vi "SVX Buffer Waterfall Graph (Plot Array).vi"(5 "reset on change to dx (F)":bool, 6 "number of spectra (40)":i32=40, 7 "reset? (F)":bool, 8 "error in (no error)":errorcluster, 9 "dz":dbl=1.0, 10 "initial z0":dbl, 11 "plots":cluster{"x0":dbl, "dx":dbl, "Y":dbl[]}[](array[cluster])) -> (0 "error out":errorcluster, 3 "waterfall graph data out":T2={"z0"=0.0, "dz"=1.0, "plots"=[]})   [LabVIEW 2017, in "SoundVib_SpectralDisplay.lvlib"]
doc: "Buffers signals and returns the buffered signals up to a maximum count. If you use this VI with the Waterfall Graph, the display mimics the behavior of a chart. Wire data to the <B>waterfall graph data</B> input to determine the polymorphic instance to use or manually select the instance."
uses:
  <vilib>/addons/Sound and Vibration/Order Analysis/Data Presentation/SoundVib_SpectralDisplay.lvlib
panel:
  in  "waterfall graph data":T1={"z0"=0.0, "dz"=1.0, "Plots"=[]}
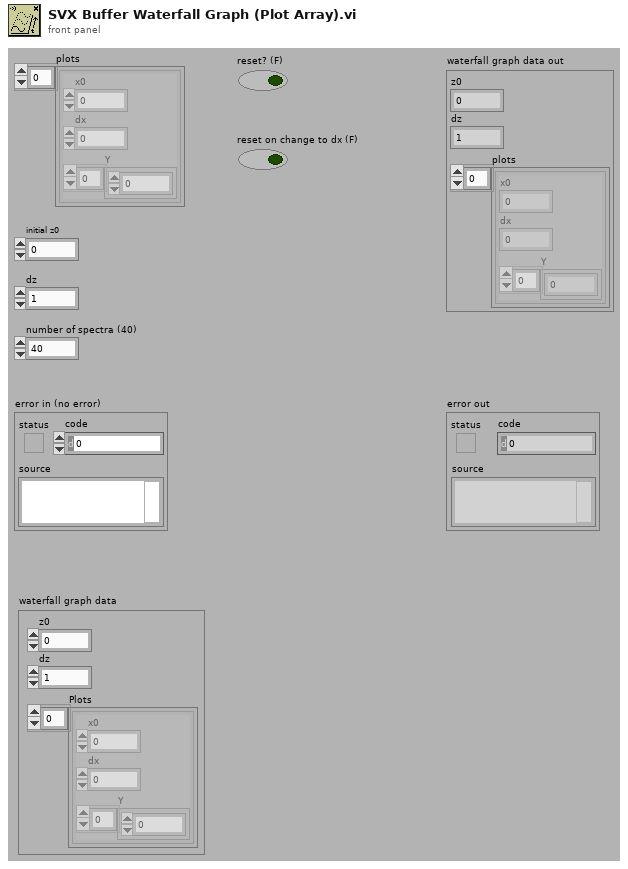
[diagram p1: front panel]
types:
  T1 = cluster{"z0":dbl, "dz":dbl, "Plots":cluster{"x0":dbl, "dx":dbl, "Y":dbl[]}[]}
  T2 = cluster{"z0":dbl, "dz":dbl, "plots":cluster{"x0":dbl, "dx":dbl, "Y":dbl[]}[]}
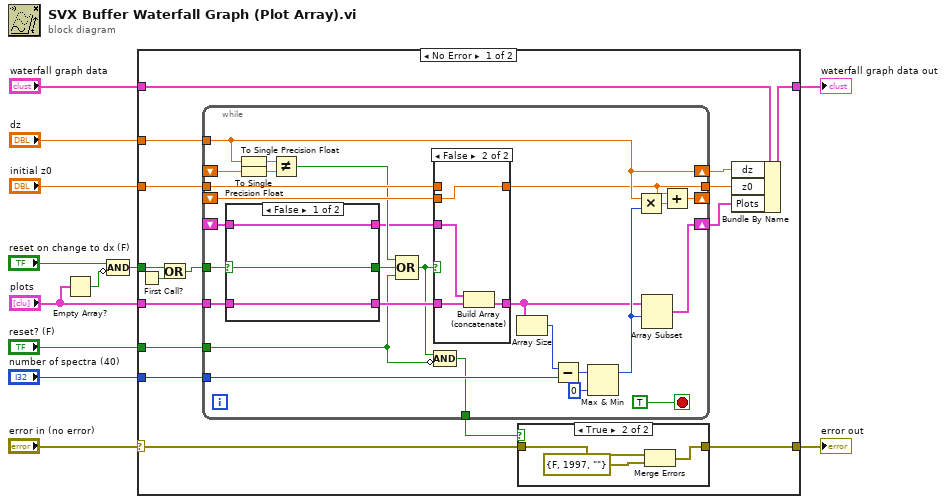
[diagram p0: block diagram]
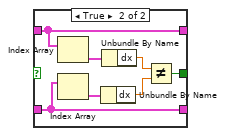
[diagram p4: hidden frame]
diagram:
  n1 = Empty Array?(array="plots") -> (empty?=w3:bool)
  n2 = Compound Arithmetic op=AND("reset on change to dx (F)", invert w3) -> (w1:bool)
  n3 = case shown="No Error" "error in (no error)" {
    selector: "error in (no error)" -> [w17 w77]
    tunnel: [w16 w77] -> w11
    tunnel: "reset? (F)" -> [w22 _]
    tunnel: "number of spectra (40)" -> [w28 _]
    tunnel: "plots" -> [w21 _]
    tunnel: [w27 w76] -> w8
    tunnel: "dz" -> [w25 _]
    tunnel: "initial z0" -> [w24 _]
    tunnel: "waterfall graph data" -> [w23 w76]
    tunnel: w1 -> [w20 _]
    frame No Error {
      n4 = First Call?() -> (First Call?: T/F=w13:bool)
      n5 = Or(x=w20, y=w13) -> (x .or. y?=w14:bool)
      n6 = while {
        tunnel: w28 -> [w41]
        shift-right: [w58] -> w26
        shift-left: _ -> [w44]
        tunnel: w22 -> [w36]
        shift-right: [w54] -> _
        shift-left: _ -> [w56]
        tunnel: w21 -> [w43]
        tunnel: w25 -> [w50]
        tunnel: w24 -> [w51]
        shift-right: [w50] -> w19
        shift-left: _ -> [w52]
        tunnel: w14 -> [w47]
        tunnel: [w35] -> w18
        tunnel: [w34] -> w15
        stop <- TRUE stop-if-true
        n7 = case shown="False" w47 {
          selector: w47 -> [w68 _]
          tunnel: w44 -> [w67 w70]
          tunnel: [w68 w73] -> w48
          tunnel: w43 -> [w66 w69]
          tunnel: [w67 w70] -> w39
          tunnel: [w66 w69] -> w40
          frame False {
          }
          frame True {
            n8 = Index Array(array=w70) -> (element=w75:cluster{"x0":dbl, "dx":dbl, "Y":dbl[]})  [unwired: 1 in]
            n9 = Index Array(array=w69) -> (element=w72:cluster{"x0":dbl, "dx":dbl, "Y":dbl[]})  [unwired: 1 in]
            n10 = Unbundle By Name(w72) -> ("dx"=w71:dbl)
            n11 = Unbundle By Name(w75) -> ("dx"=w74:dbl)
            n12 = Not Equal?(x=w74, y=w71) -> (x != y?=w73:bool)
          }
        }
        n13 = To Single Precision Float(number=w50) -> (single precision float=w45:sgl)
        n14 = To Single Precision Float(number=w52) -> (single precision float=w46:sgl)
        n15 = Not Equal?(x=w45, y=w46) -> (x != y?=w49:bool)
        n16 = Compound Arithmetic op=OR(w49, w48, w36) -> (w37:bool)
        n17 = case shown="False" w37 {
          tunnel: [w60 w62] -> w33
          tunnel: w56 -> [_ w65]
          tunnel: [w61 w65] -> w34
          tunnel: w51 -> [w61 _]
          tunnel: w39 -> [_ w63]
          tunnel: w40 -> [w60 w64]
          frame True {
          }
          frame False {
            n18 = Build Array (concatenate)(w63, w64) -> (w62:cluster{"x0":dbl, "dx":dbl, "Y":dbl[]}[])
          }
        }
        n19 = Compound Arithmetic op=AND(w37, invert w36) -> (w35:bool)
        n20 = Array Size(array=w33) -> (size(s)=w42:i32)
        n21 = Subtract(x=w42, y=w41) -> (x-y=w38:i32)
        n22 = Max & Min(x=w38, y=0) -> (max(x,y)=w53:i32)  [unwired: 1 out]
        n23 = Multiply(x=w50, y=w53) -> (x*y=w55:dbl)
        n24 = Array Subset(array=w33, index=w53) -> (w58:cluster{"x0":dbl, "dx":dbl, "Y":dbl[]}[])  [unwired: 1 in]
        n25 = Add(x=w34, y=w55) -> (x+y=w54:dbl)
      }
      n26 = case shown="True" w18 {
        tunnel: w17 -> [w29 w31]
        tunnel: [w29 w32] -> w16
        frame False {
        }
        frame True {
          n27 = Merge Errors(w31, errorcluster {"status"=FALSE, "code"=1997, "source"=""} ("error in 2 (no error)")) -> (w32:errorcluster)
        }
      }
      n28 = Bundle By Name(cluster=w23, "dz"=w19, "z0"=w15, "Plots"=w26) -> (w27:T1)
    }
    frame Error {
    }
  }
  "waterfall graph data out" <- w8
  "error out" <- w11
